vi "stateMachineAutomatic.vi"() -> ()   [LabVIEW 2019]
uses:
  EnumSt.ctl
panel:
  in  "Time":u32
  out "LostTime":u32
  out "Waveform Chart":cluster{"number: 0 to 1":dbl, "res":dbl}(graph)
  in  "stop":bool
  in  "State":T1
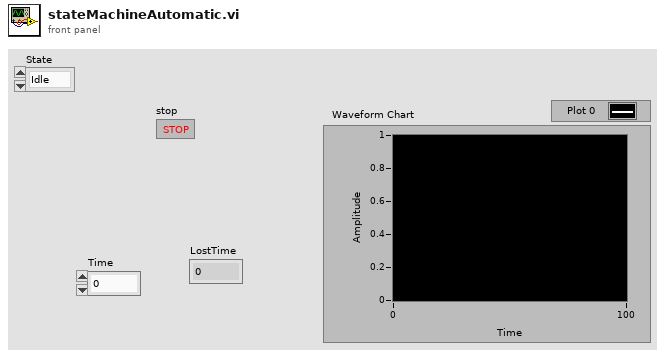
[diagram p1: front panel]
types:
  T1 = typedef "EnumSt.ctl" = enum16{"Idle", "Merch", "Analyze", "Stop"}
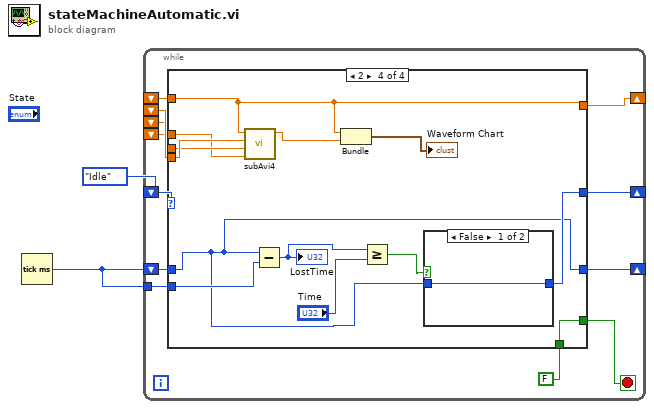
[diagram p0: block diagram]
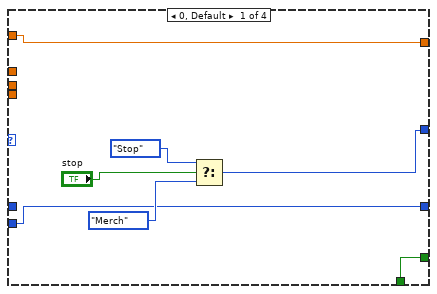
[diagram p2: hidden frame]
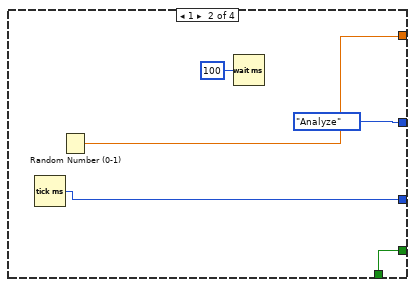
[diagram p3: hidden frame]
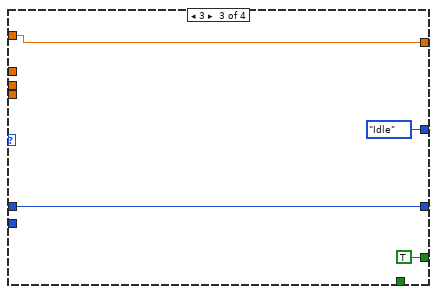
[diagram p4: hidden frame]
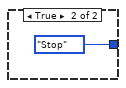
[diagram p5: hidden frame]
diagram:
  n1 = Tick Count (ms)() -> (millisecond timer value=w1:u32)
  n2 = while {
    shift-right: [w13] -> _
    shift-left: EnumSt."Idle" ("State") -> [w14]
    shift-right: [w10] -> _
    shift-left: _ -> [w9]
    shift-left: _ -> [w8]
    shift-left: _ -> [w7]
    shift-left: _ -> [w6]
    shift-right: [w4] -> _
    shift-left: w1 -> [w5]
    tunnel: w1 -> [w3]
    stop <- w12 stop-if-true
    n3 = case shown="2" w14 {
      tunnel: [w16 EnumSt."Analyze" ("State") EnumSt."Idle" ("State") w32] -> w13
      tunnel: [w21 w24 TRUE w38] -> w12
      tunnel: FALSE -> [w21 w24 _ w38]
      tunnel: [w20 w26 w28 w37] -> w10
      tunnel: w9 -> [w20 _ w28 w37]
      tunnel: w8 -> [_ _ _ w43]
      tunnel: w7 -> [_ _ _ w42]
      tunnel: w6 -> [_ _ _ w41]
      tunnel: w5 -> [_ _ w27 w31]
      tunnel: [w15 w22 w27 w31] -> w4
      tunnel: w3 -> [w15 _ _ w36]
      frame 0, Default {
        n4 = Select(t=EnumSt."Stop" ("State"), s="stop", f=EnumSt."Merch" ("State")) -> (s? t:f=w16:T1)
      }
      frame 1 {
        n5 = Tick Count (ms)() -> (millisecond timer value=w22:u32)
        n6 = Random Number (0-1)() -> (number: 0 to 1=w26:dbl)
        n7 = Wait (ms)(milliseconds to wait=u32 100) -> ()  [unwired: 1 out]
      }
      frame 3 {
      }
      frame 2 {
        n8 = call "subAvi4.vi"("Numeric 4"=w41, "Numeric 3"=w42, "Numeric 2"=w43, "Numeric"=w37) -> ("res"=w40:dbl)  [unwired: 7 in]
        n9 = Subtract(x=w31, y=w36) -> (x-y=w35:u32)
        "LostTime" <- w35
        n10 = Bundle("number: 0 to 1"=w37, "res"=w40) -> (→"Waveform Chart":cluster{"number: 0 to 1":dbl, "res":dbl})  [unwired: 1 in]
        n11 = Greater Or Equal?(x=w35, y="Time") -> (x >= y?=w33:bool)
        n12 = case shown="False" w33 {
          tunnel: [w44 EnumSt."Stop" ("State")] -> w32
          tunnel: w31 -> [w44 _]
          frame False {
          }
          frame True {
          }
        }
      }
    }
  }
